vi "Valve-Main.vi"(8 "error In":errorcluster) -> (0 "error out":errorcluster)   [LabVIEW 2021]
doc: "Use this template to build a simple state machine design pattern. Each state executes code and determines which state to transition to."
uses:
  Controls/Valve-State.ctl
  Controls/Valve-Data.ctl
  Valve-Module.lvlib
panel:
  out "Status":string
  in  "Valve 3":bool
  in  "Valve 2":bool
  in  "Valve 1":bool
  out "V 3":bool
  out "V 2":bool
  out "V 1":bool
  in  "Fire Valves":bool
  in  "Exit":bool
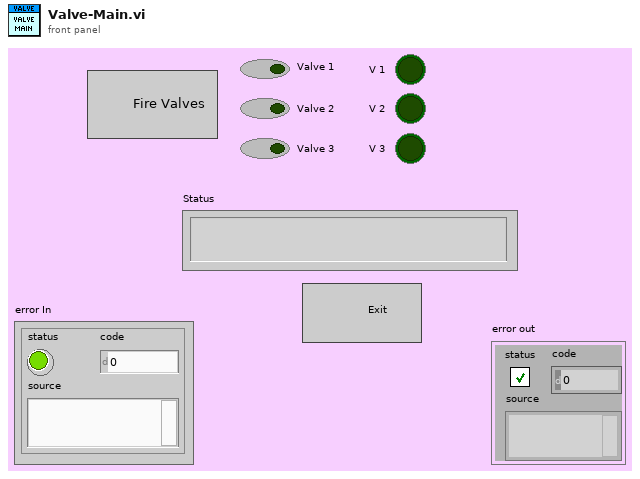
[diagram p1: front panel]
types:
  T1 = typedef "Valve-Data.ctl" = cluster{"Fire":bool, "Status":string, "Valves":bool[]}
  T2 = typedef "Valve-State.ctl" = enum16{"Initialize", "Wait for Event", "Valves: Fire", "Do: Nothing", "Exit"}
  T3 = typedef "Valve-Module.lvlib/Request Events--cluster.ctl" = cluster{"Stop":refnum<user-event>, "Write Fire Valves":refnum<user-event>}
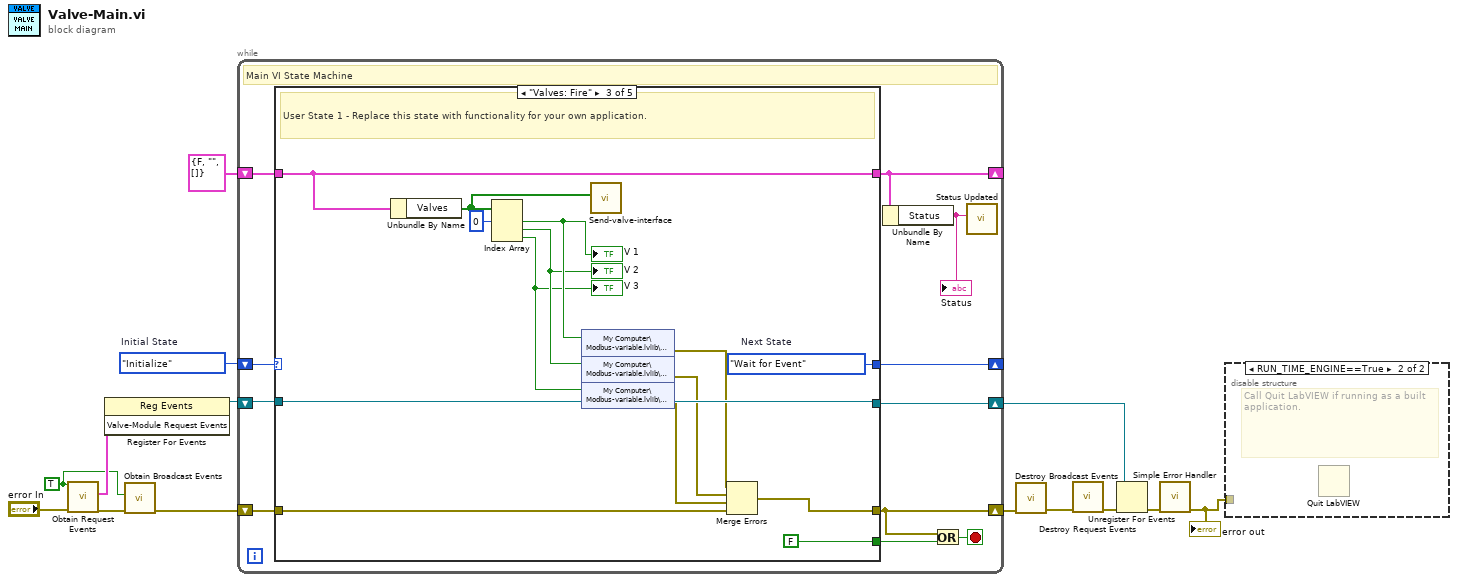
[diagram p0: block diagram]
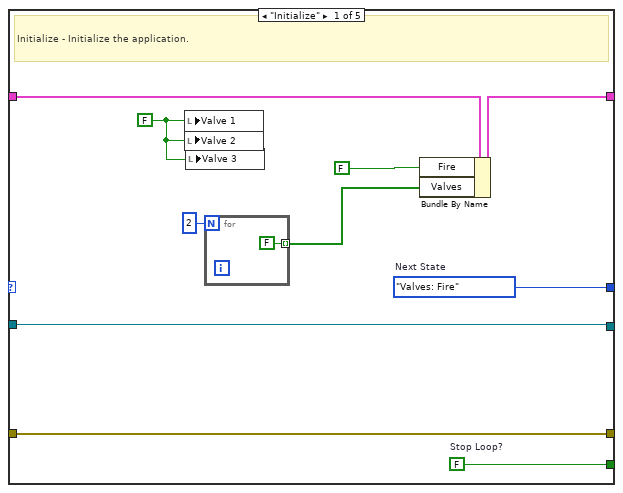
[diagram p3: hidden frame]
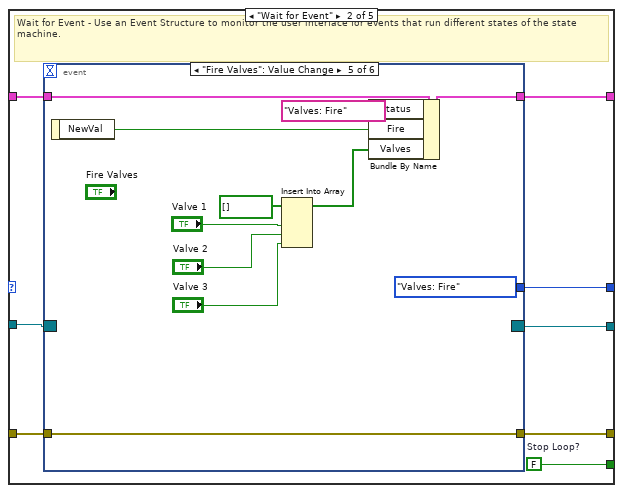
[diagram p4: hidden frame]
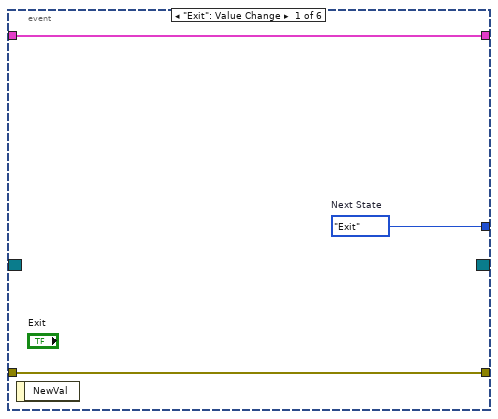
[diagram p5: hidden frame]
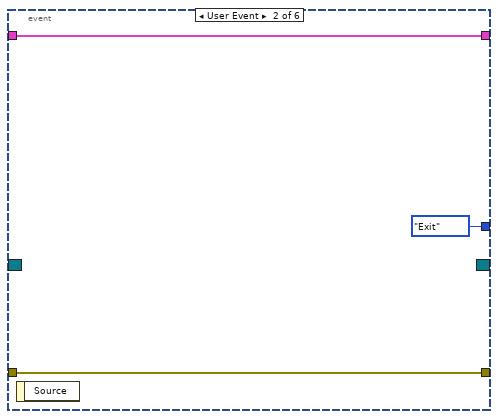
[diagram p6: hidden frame]
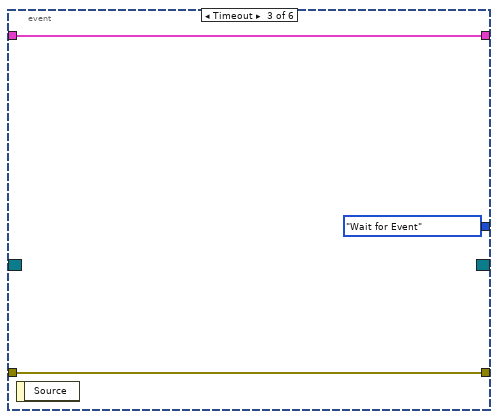
[diagram p7: hidden frame]
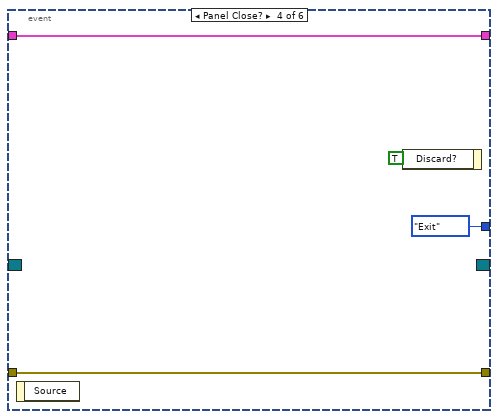
[diagram p8: hidden frame]
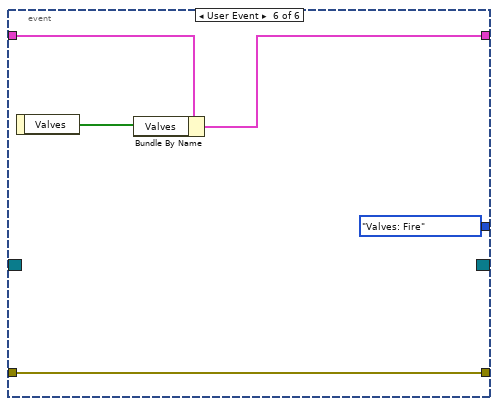
[diagram p9: hidden frame]
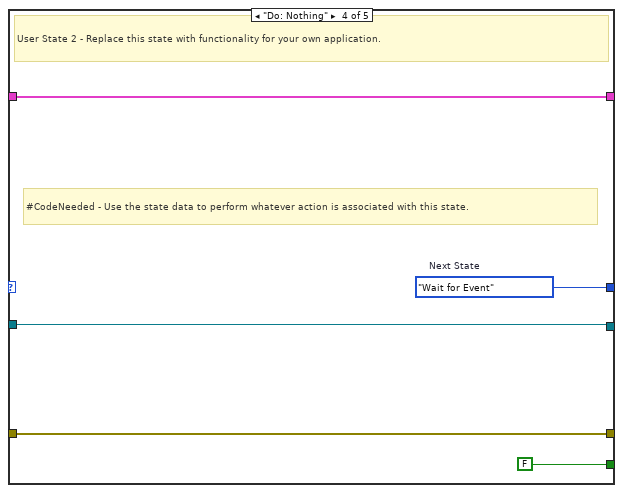
[diagram p10: hidden frame]
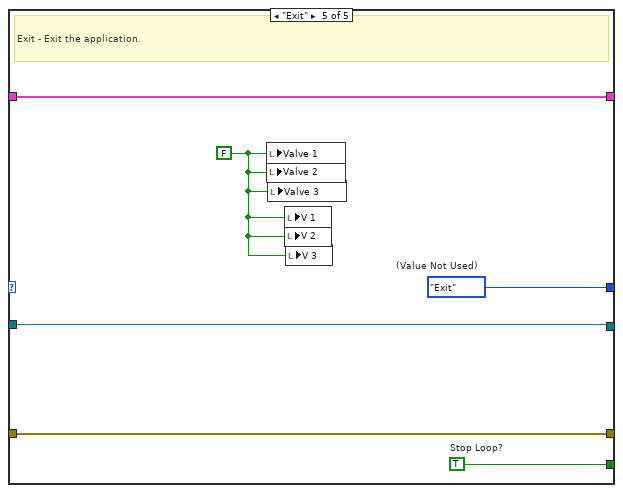
[diagram p11: hidden frame]
diagram:
  w6 = TRUE ("Create New?")
  w14 = Valve-State."Initialize"  # Initial State
  n1 = call "Obtain Request Events.vi"("error in (no error)"="error In", "Create New?"=w6) -> ("error out"=w11:errorcluster, "Valve-Module Request Events"=w8:T3)  [unwired: 8 in]
  n2 = register-events(w8) -> (reference out=w7:refnum<event-registration>)  [unwired: 2 in, 1 out]
  n3 = call "Obtain Broadcast Events.vi"("error in (no error)"=w11, "Create New?"=w6) -> ("error out"=w9:errorcluster)  [unwired: 8 in, 1 out]
  n4 = while {
    shift-right: [w24] -> _
    shift-left: w14 -> [w25]
    shift-right: [w16] -> _
    shift-left: T1 {"Fire"=FALSE, "Status"="", "Valves"=[]} ("Data") -> [w23]
    shift-right: [w19] -> w4
    shift-left: w9 -> [w22]
    shift-right: [w17] -> w1
    shift-left: w7 -> [w18]
    stop <- w20 stop-if-true
    # "Main VI State Machine"
    n5 = case shown="\"Valves: Fire\"" w25 {
      tunnel: [w35 w44 w87 w92 w98] -> w24
      tunnel: [w34 w43 FALSE ("Stop Loop?") FALSE ("Stop Loop?") w96] -> w21
      tunnel: w23 -> [w33 w42 w85 w90 w97]
      tunnel: [w32 w41 w85 w90 w97] -> w16
      tunnel: w22 -> [w30 w40 w84 w89 w95]
      tunnel: [w30 w39 w77 w89 w95] -> w19
      tunnel: w18 -> [w29 w38 w83 w88 w94]
      tunnel: [w29 w37 w83 w88 w94] -> w17
      frame "Initialize" {
        w26 = FALSE ("Valve 1")
        w34 = FALSE  # Stop Loop?
        w35 = Valve-State."Valves: Fire"  # Next State
        # "Initialize - Initialize the application."
        n6 = local write "Valve 1"(w26) -> ()
        n7 = local write "Valve 2"(w26) -> ()
        n8 = local write "Valve 3"(w26) -> ()
        n9 = for {
          N: 2 -> [_]
          tunnel: [FALSE] -> w27 mode=indexing
        }
        n10 = Bundle By Name(cluster=w33, "Fire"=FALSE ("Replace_Me_Boolean"), "Valves"=w27) -> (w32:T1)
      }
      frame "Wait for Event" {
        w43 = FALSE  # Stop Loop?
        # "Wait for Event - Use an Event Structure to monitor the user interface for events that run different states of the state machine."
        n11 = event shown="[4] \"Fire Valves\": Value Change" {
          selector: w38 -> [_ _ _ _ _ _]
          dyn-events: [_ _ _ _ _ _] -> w37
          timeout: _ -> [_ _ _ _ _ _]
          tunnel: [w47 Valve-State."Exit" ("Next State") Valve-State."Wait for Event" ("Next State") Valve-State."Exit" ("Next State") Valve-State."Valves: Fire" ("Next State") Valve-State."Valves: Fire" ("Next State")] -> w44
          tunnel: w42 -> [w46 w50 w53 w57 w68 w70]
          tunnel: [w46 w50 w53 w57 w67 w69] -> w41
          tunnel: w40 -> [w45 w49 w52 w56 w66 w73]
          tunnel: [w45 w49 w52 w56 w66 w73] -> w39
          event "Exit": Value Change {
            w47 = Valve-State."Exit"  # Next State
            n12 = event-data() -> ()  [unwired: 1 in, 1 out]
          }
          event User Event {
            n13 = event-data() -> ()  [unwired: 1 in, 1 out]
          }
          event Timeout {
            n14 = event-data() -> ()  [unwired: 1 in, 1 out]
          }
          event Panel Close? {
            n15 = event-data() -> ()  [unwired: 1 in, 1 out]
            n16 = event-data("Discard?"=TRUE) -> ()  [unwired: 1 in, 1 out]
          }
          event "Fire Valves": Value Change {
            n17 = event-data() -> ("NewVal"=w63:bool)  [unwired: 1 in]
            n18 = Insert Into Array(array=bool[] [], new element #1="Valve 1", new element #2="Valve 2", new element #3="Valve 3") -> (w58:bool[])  [unwired: 1 in]
            n19 = Bundle By Name(cluster=w68, "Status"="Valves: Fire", "Fire"=w63, "Valves"=w58) -> (w67:T1)
          }
          event User Event {
            n20 = event-data() -> ("Valves"=w71:bool[])  [unwired: 1 in]
            n21 = Bundle By Name(cluster=w70, "Valves"=w71) -> (w69:T1)
          }
        }
      }
      frame "Valves: Fire" {
        w87 = Valve-State."Wait for Event"  # Next State
        # "User State 1 - Replace this state with functionality for your own application."
        n22 = Unbundle By Name(w85) -> ("Valves"=w81:bool[])
        n23 = Index Array(array=w81, index #1=0 ("index")) -> (element #1=w80:bool, element #2=w79:bool, element #3=w78:bool)  [unwired: 2 in]
        "V 1" <- w80
        "V 2" <- w79
        "V 3" <- w78
        n24 = shared-variable "My Computer\\Modbus-variable.lvlib\\000049"(w80) -> (error out=w76:errorcluster)  [unwired: 1 in]
        n25 = shared-variable "My Computer\\Modbus-variable.lvlib\\000050"(w79) -> (error out=w75:errorcluster)  [unwired: 1 in]
        n26 = shared-variable "My Computer\\Modbus-variable.lvlib\\000051"(w78) -> (error out=w74:errorcluster)  [unwired: 1 in]
        n27 = call "Send-valve-interface.vi"("Valves"=w81) -> ()  [unwired: 10 in, 1 out]
        n28 = Merge Errors(w76, w75, w74, w84) -> (w77:errorcluster)
      }
      frame "Do: Nothing" {
        w92 = Valve-State."Wait for Event"  # Next State
        # "#CodeNeeded - Use the state data to perform whatever action is associated with this state."
        # "User State 2 - Replace this state with functionality for your own application."
      }
      frame "Exit" {
        w93 = FALSE ("Valve 1")
        w96 = TRUE  # Stop Loop?
        w98 = Valve-State."Exit"  # (Value Not Used)
        # "Exit - Exit the application."
        n29 = local write "Valve 1"(w93) -> ()
        n30 = local write "Valve 2"(w93) -> ()
        n31 = local write "Valve 3"(w93) -> ()
        n32 = local write "V 1"(w93) -> ()
        n33 = local write "V 2"(w93) -> ()
        n34 = local write "V 3"(w93) -> ()
      }
    }
    n35 = Unbundle By Name(w16) -> ("Status"=w15:string)
    "Status" <- w15
    n36 = Or(x=w19, y=w21) -> (x .or. y?=w20:bool)
    n37 = call "Status Updated.vi"("Status"=w15) -> ()  [unwired: 10 in, 1 out]
  }
  n38 = call "Destroy Broadcast Events.vi"("error in (no error)"=w4) -> ("error out"=w5:errorcluster)  [unwired: 10 in]
  n39 = call "Destroy Request Events.vi"("error in (no error)"=w5) -> ("error out"=w3:errorcluster)  [unwired: 10 in]
  n40 = Unregister For Events(event registration refnum=w1, error in=w3) -> (error out=w2:errorcluster)
  n41 = call <vilib>:"Simple Error Handler.vi"("error in (no error)"=w2) -> ("error out"=w12:errorcluster)  [unwired: 4 in, 4 out]
  "error out" <- w12
  n42 = disable-structure shown="RUN_TIME_ENGINE==True" {
    disable-tunnel: w12 -> [_ _]
    frame condition #0 (active) {
    }
    frame condition #1 {
      # "Call Quit LabVIEW if running as a built application."
      n43 = Quit LabVIEW() -> ()  [unwired: 1 in]
    }
  }
